vi "test Initialize Engine Pointer.vi"(8 "error in (no error)":errorcluster, 11 "TestCase in":refnum<class "Framework Tests.lvclass">) -> (0 "error out":errorcluster, 3 "TestCase out":refnum<class "Framework Tests.lvclass">)   [LabVIEW 2017, in "Framework Tests.lvclass"]
uses:
  Framework Tests.lvclass
  Engine/Classes/Framework/Framework.lvclass
  <vilib>/NI/Memory Manager/Classes/Pointer/Pointer.lvclass/Pointer.ctl
  Engine/Classes/Framework/Framework.lvclass/Framework.ctl
  <vilib>/NI/Memory Manager/Classes/Pointer/Public/New/New (1B).vi
  <vilib>/NI/Memory Manager/Classes/Pointer/Public/Write/Write (0D Bool).vi
  <vilib>/NI/Memory Manager/Classes/Pointer/Public/Read/Read (0D Bool).vi
  <vilib>/NI/Memory Manager/Classes/Pointer/Private/Allocate.vi
  <vilib>/NI/Memory Manager/Classes/Pointer/Public/Write (No Check)/Write (No Check 0D Bool).vi
  <vilib>/NI/Memory Manager/Classes/Pointer/Protected/Parameter Checking/Check Null Pointer.vi
  <vilib>/NI/Memory Manager/Classes/Pointer/Protected/Parameter Checking/Check Subset.vi
  <vilib>/NI/Memory Manager/Classes/Pointer/Public/Read (No Check)/Read (No Check 0D Bool).vi
  <vilib>/NI/Memory Manager/Classes/Pointer/API/Accessors/Set Address.vi
  <vilib>/NI/Memory Manager/Classes/Pointer/API/Accessors/Set Size.vi
  <vilib>/NI/Memory Manager/Classes/Pointer/Private/Set Internal.vi
  <vilib>/NI/Memory Manager/Classes/Pointer/API/Accessors/Get Address.vi
  <vilib>/NI/Memory Manager/Classes/Pointer/Protected/Errors.vi
  <vilib>/NI/Memory Manager/Classes/Pointer/Protected/Error VIs/Null Pointer.vi
  <vilib>/NI/Memory Manager/Classes/Pointer/Protected/Error VIs/Out of Bounds.vi
  <vilib>/NI/Memory Manager/Classes/Pointer/API/Accessors/Get Size.vi
  <vilib>/NI/Memory Manager/Classes/Pointer/Protected/Error Building/Create Error.vi
  <vilib>/NI/Memory Manager/VIs/Write String into Source.vi
  <vilib>/NI/Memory Manager/Classes/Pointer/Protected/Error Building/Write Pointer Size.vi
  <vilib>/NI/Memory Manager/VIs/Write Number into Source.vi
  <vilib>/NI/Memory Manager/VIs/VIs for Poly/Write U64 into Source.vi
  <vilib>/NI/Memory Manager/Constants/Constants.vi
  <vilib>/NI/Memory Manager/Constants/Library Name.vi
  <vilib>/NI/Memory Manager/Classes/Pointer/Protected/Error Building/Get Error Info.vi
  <vilib>/NI/Memory Manager/VIs/Create Error Cluster.vi
  <vilib>/NI/Memory Manager/VIs/VIs for Poly/Create Error Cluster (256B).vi
  <vilib>/NI/Memory Manager/VIs/Set Error Status.vi
  <vilib>/NI/Memory Manager/VIs/Set Error Code.vi
  <vilib>/NI/Memory Manager/VIs/Set Error Source.vi
  <vilib>/NI/Memory Manager/Classes/Pointer/Pointer.lvclass
  <vilib>/addons/_JKI Toolkits/VI Tester/TestCase.llb/TestCase.lvclass
  C:/Program Files (x86)/National Instruments/LabVIEW 2017/vi.lib/addons/_JKI Toolkits/VI Tester/TestCase.llb/TestCase.lvclass
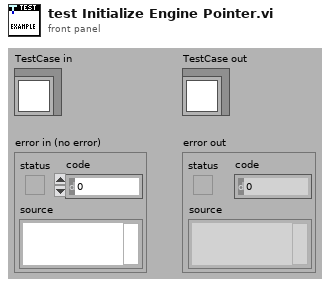
[diagram p1: front panel]
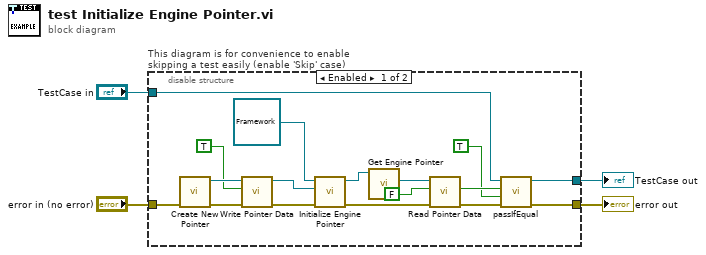
[diagram p0: block diagram]
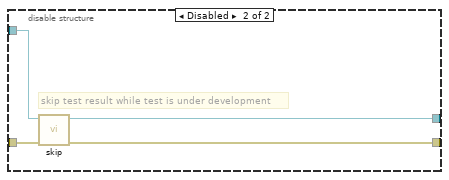
[diagram p2: hidden frame]
diagram:
  n1 = disable-structure "This diagram is for convenience to enable skipping a test easily (enable 'Skip' case)" shown="Enabled" {
    disable-tunnel: "TestCase in" -> [w8 w25]
    disable-tunnel: [w7 w23] -> w1
    disable-tunnel: [w9 w24] -> w3
    disable-tunnel: "error in (no error)" -> [w14 w22]
    frame Enabled {
      n2 = call-poly <vilib>:"Create New Pointer.vi"("error in (no error)"=w14) -> ("error out"=w13:errorcluster, "Pointer"=w20:refnum<class "Pointer.lvclass">)  [unwired: 9 in]
      n3 = call-poly <vilib>:"Write Pointer Data.vi"("error in (no error)"=w13, "value"=TRUE, "Pointer in"=w20) -> ("error out"=w12:errorcluster, "Pointer out"=w19:refnum<class "Pointer.lvclass">)  [unwired: 5 in, 2 out]
      n4 = call "Initialize Engine Pointer.vi"("error in (no error)"=w12, "Engine Pointer"=w19, "Framework in"=refnum<class "Framework.lvclass"> refnum) -> ("error out"=w11:errorcluster, "Framework out"=w17:refnum<class "Framework.lvclass">)  [unwired: 7 in]
      n5 = call "Get Engine Pointer.vi"("Framework in"=w17) -> ("Engine Pointer"=w16:refnum<class "Pointer.lvclass">)  [unwired: 9 in, 1 out]
      n6 = call-poly <vilib>:"Read Pointer Data.vi"("error in (no error)"=w11, "value in"=FALSE, "Pointer in"=w16) -> ("error out"=w10:errorcluster, "value out"=w6:bool)  [unwired: 5 in, 2 out]
      n7 = call-dynamic "passIfEqual.vi"("error in (no error)"=w10, "y"=TRUE ("value out"), "x"=w6, "TestCase in"=w8) -> ("error out"=w9:errorcluster, "TestCase out"=w7:refnum<class "Framework Tests.lvclass">)  [unwired: 6 in]
    }
    frame Disabled {
      # "skip test result while test is under development"
      n8 = call <vilib>:"skip.vi"("error in (no error)"=w22, "TestCase in"=w25) -> ("error out"=w24:errorcluster, "TestCase out"=w23:refnum<class "Framework Tests.lvclass">)  [unwired: 8 in]
    }
  }
  "error out" <- w3
  "TestCase out" <- w1
